vi "ExtractingCSVdata.vi"() -> ()   [LabVIEW 2020]
uses:
  <vilib>/Utility/file.llb/Read Delimited Spreadsheet (DBL).vi
panel:
  out "Voltage_0 (V)":dbl[](array[numeric])
  out "Displacement sensor output (V)":dbl[](array[numeric])
  out "Time (ms)":dbl[](array[numeric])
  in  "file path (dialog if empty)":path
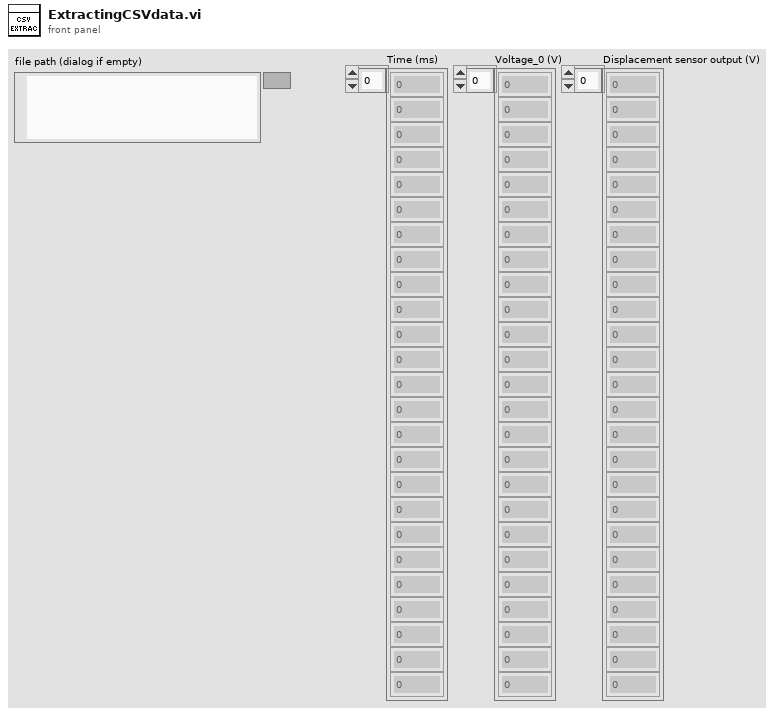
[diagram p1: front panel]
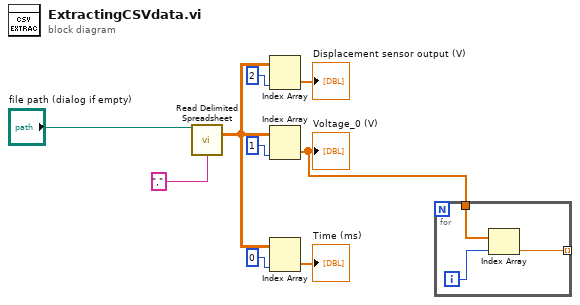
[diagram p0: block diagram]
diagram:
  n1 = call-poly <vilib>:"Read Delimited Spreadsheet.vi"("file path (dialog if empty)"="file path (dialog if empty)", "delimiter (\\t)"="," ("delimiter (\\t)")) -> ("all rows"=w2:dbl[][])  [unwired: 8 in, 5 out]
  n2 = Index Array(array=w2, index (col)=2 ("disabled index (col)")) -> (element=→"Displacement sensor output (V)":dbl[])  [unwired: 1 in]
  n3 = Index Array(array=w2, index (col)=1 ("disabled index (col)")) -> (element=w1:dbl[])  [unwired: 1 in]
  "Voltage_0 (V)" <- w1
  n4 = Index Array(array=w2, index (col)=0 ("disabled index (col)")) -> (element=→"Time (ms)":dbl[])  [unwired: 1 in]
  n5 = for {
    tunnel: w1 -> [w12]
    tunnel: [w10] -> _ mode=indexing
    i -> [w11]
    n6 = Index Array(array=w12, index=w11) -> (element=w10:dbl)
  }
